vi "Actor Core.vi"(8 "error in":errorcluster, 11 "Sensor in":refnum<class "Sensor.lvclass">) -> (0 "error out":errorcluster, 3 "Actor out":refnum<class "Actor.lvclass">)   [LabVIEW 2020, in "Sensor.lvlib" / "Sensor.lvclass"]
doc: "(<B>Filename</B>: Actor Framework.lvlib:Actor.lvclass:Actor Core.vi)\n\nReceives messages to the actor, reacts to them, and initiates any error handling that may shut the actor down.\n\nDescendant classes may override this VI to append parallel tasks for the actor to complete while it handles messages. Overrides use the Call Parent Class Method node."
uses:
  Sensor.lvclass
  <vilib>/ActorFramework/Actor/Actor.lvclass
  Sensor.lvclass/Sensor.ctl
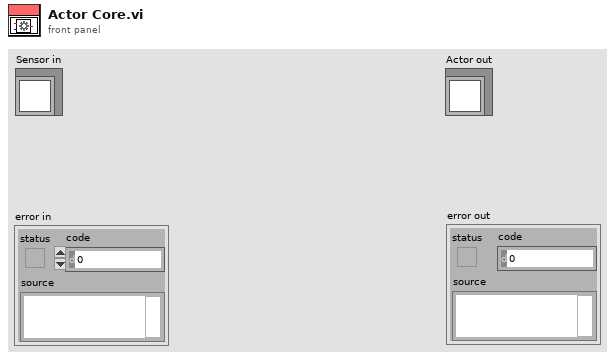
[diagram p1: front panel]
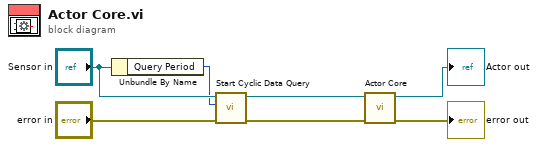
[diagram p0: block diagram]
diagram:
  n1 = Unbundle By Name("Sensor in") -> ("Query Period"=w1:i32)
  n2 = call-dynamic "Start Cyclic Data Query.vi"("error in (no error)"="error in", "Query Period (ms)"=w1, "Sensor in"="Sensor in") -> ("error out"=w4:errorcluster, "Sensor out"=w5:refnum<class "Sensor.lvclass">)  [unwired: 7 in]
  n3 = call-parent "Actor Core.vi"("error in"=w4, "Actor in"=w5) -> ("error out"=→"error out":errorcluster, "Actor out"=→"Actor out":refnum<class "Actor.lvclass">)  [unwired: 8 in]
